vi "Add_LDA_Probe_Type.vi"() -> (0 "Cancel Out":bool, 1 "New LDA Probe Type Out":T1)   [LabVIEW 2010]
panel:
  in  "Cancel Button":bool
  in  "OK":bool
  in  "New LDA Probe Type":T1
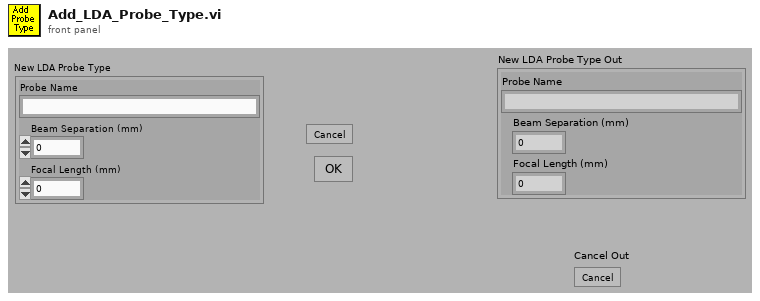
[diagram p1: front panel]
types:
  T1 = cluster{"Probe Name":string, "Beam Separation (mm)":dbl, "Focal Length (mm)":dbl}
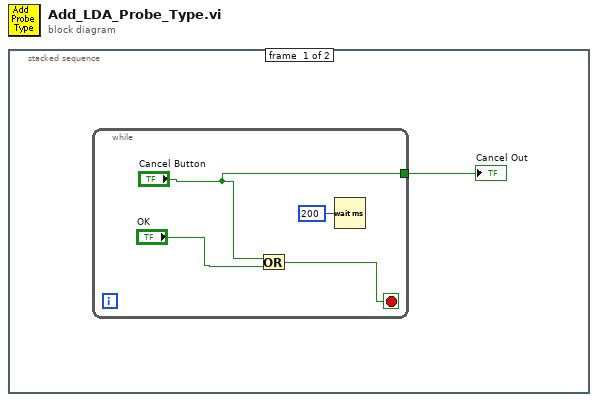
[diagram p0: block diagram]
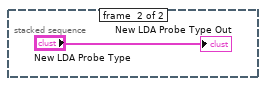
[diagram p2: hidden frame]
diagram:
  n1 = stacked-sequence {
    frame #0 {
      n2 = while {
        tunnel: ["Cancel Button"] -> w1
        stop <- w4 stop-if-true
        n3 = Or(x="Cancel Button", y="OK") -> (x .or. y?=w4:bool)
        n4 = Wait (ms)(milliseconds to wait=u32 200) -> ()  [unwired: 1 out]
      }
      "Cancel Out" <- w1
    }
    frame #1 {
      "New LDA Probe Type Out" <- "New LDA Probe Type"
    }
  }
